vi "Serialize - JSON.vi"(8 "error in":errorcluster, 11 "Data in":refnum<class "Data.lvclass">) -> (0 "error out":errorcluster, 2 "Serialized JSON":string, 3 "Data out":refnum<class "Data.lvclass">)   [LabVIEW 2016, in "Base Data Class.lvlib" / "Data.lvclass"]
uses:
  Data.lvclass
  Data.lvclass/Data.ctl
  Read Data ID.vi
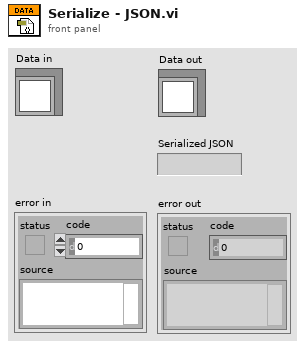
[diagram p1: front panel]
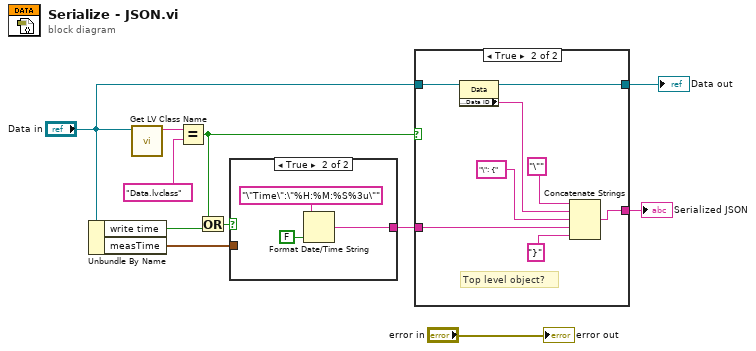
[diagram p0: block diagram]
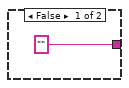
[diagram p3: hidden frame]
diagram:
  n1 = Unbundle By Name("Data in") -> ("write time"=w7:bool, "measTime"=w10:timestamp)
  n2 = call <vilib>:"Get LV Class Name.vi"("object"="Data in") -> ("class name"=w9:string)  [unwired: 9 in, 1 out]
  n3 = Equal?(x=w9, y="Data.lvclass") -> (x = y?=w5:bool)
  n4 = Or(x=w5, y=w7) -> (x .or. y?=w6:bool)
  n5 = case shown="True" w6 {
    tunnel: w10 -> [_ _]
    tunnel: ["" w13] -> w3
    frame False {
    }
    frame True {
      n6 = Format Date/Time String(time format string (%c)="\"Time\":\"%H:%M:%S%3u\"", UTC format=FALSE) -> (date/time string=w13:string)  [unwired: 1 in]
    }
  }
  n7 = case shown="True" w5 {
    tunnel: "Data in" -> [w16 w25]
    tunnel: w3 -> [w17 w21]
    tunnel: [w17 w19] -> w2
    tunnel: [w16 w18] -> w1
    frame False {
    }
    frame True {
      # "Top level object?"
      n8 = property class="Data"(reference=w25) -> (reference out=w18:refnum<class "Data.lvclass">, "Accessors:Data ID"=w24:string)  [unwired: 1 in, 1 out]
      n9 = Concatenate Strings("\"" ("string"), w24, "\": {" ("string"), w21, "}" ("string")) -> (w19:string)
    }
  }
  "Data out" <- w1
  "Serialized JSON" <- w2
  "error out" <- "error in"
